vi "Main.vi"() -> ()   [LabVIEW 2019, in "gRPC Scripting Tools.lvlib"]
uses:
  gRPC Scripting Tools.lvlib
  TypeDefs/Project Settings.ctl
panel:
  in  "Generate":enum16{"gRPC Server", "gRPC Client", "Both"}(ring)
  in  "Target Name":string
  in  "Generated Library Name (\"_server\" / \"_client\" will be auto appended)":string
  in  "Target Project":path
  in  "Proto File Path":path
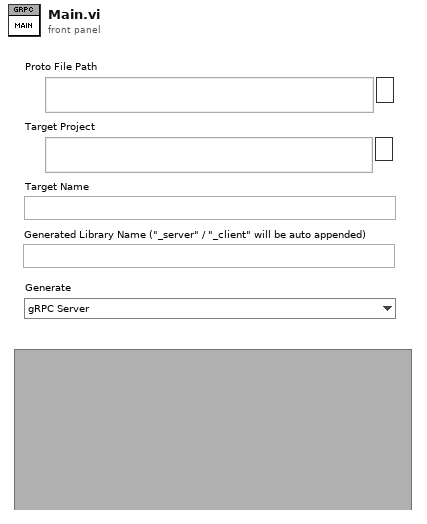
[diagram p1: front panel]
types:
  T1 = typedef "gRPC Scripting Tools.lvlib/RPC Method Parameters.ctl" = cluster{"RPC Method Name":string, "Request Metadata Name":string, "Response Metadata Name":string, "Client Streaming":bool, "Server Streaming":bool}
  T2 = typedef "gRPC Scripting Tools.lvlib/Message Metadata (Scripting).ctl" = cluster{"Version":i32, "Name":string, "Type Url":string, "Elements":T3[]}
  T3 = typedef "gRPC Scripting Tools.lvlib/Message Element Metadata (Scripting).ctl" = cluster{"Field Name":string, "Embedded Message Name":string, "Protobuf Index":i32, "MessageElementType":T4, "Repeated":bool}
  T4 = typedef "gRPC Scripting Tools.lvlib/Message Element Type.ctl" = enum32{"Int32Value", "FloatValue", "DoubleValue", "BoolValue", "StringValue", "MessageValue", "Int64Value", "UInt32Value", "UInt64Value", "EnumValue", "Bytes", "Fixed64", "Fixed32", "SFixed64", "SFixed32", "SInt64", "SInt32"}
  T5 = typedef "gRPC Scripting Tools.lvlib/Project Settings.ctl" = cluster{"Target Project Path":path, "Target Name":string, "Server Name":string, "Library Path":path}
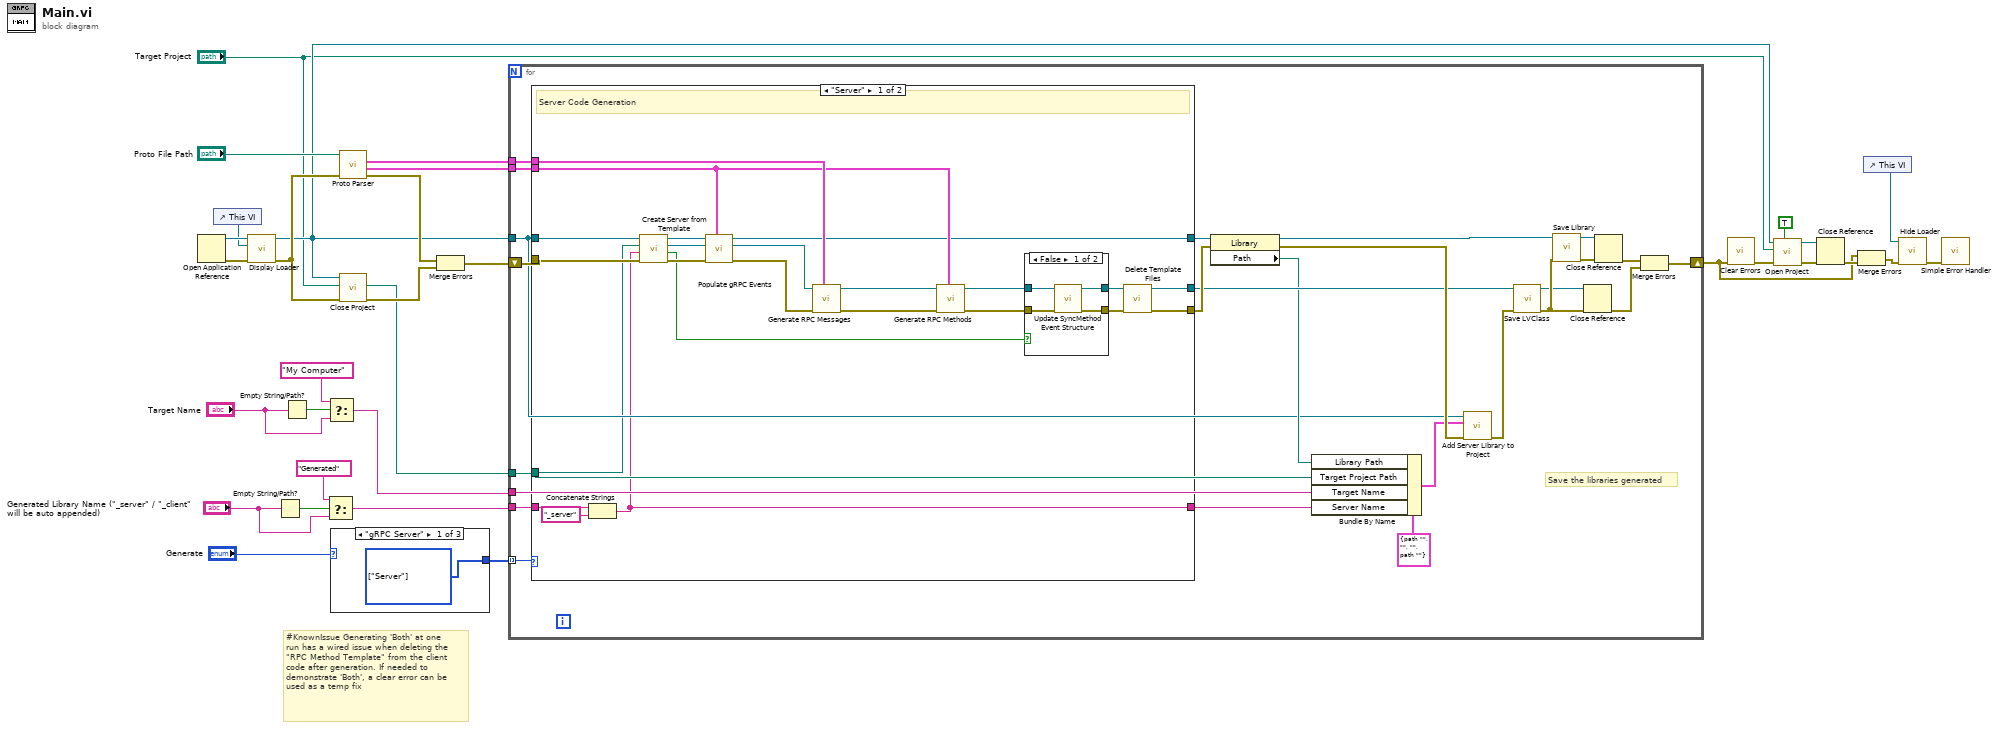
[diagram p0: block diagram]
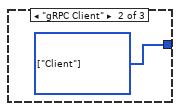
[diagram p2: hidden frame]
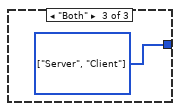
[diagram p3: hidden frame]
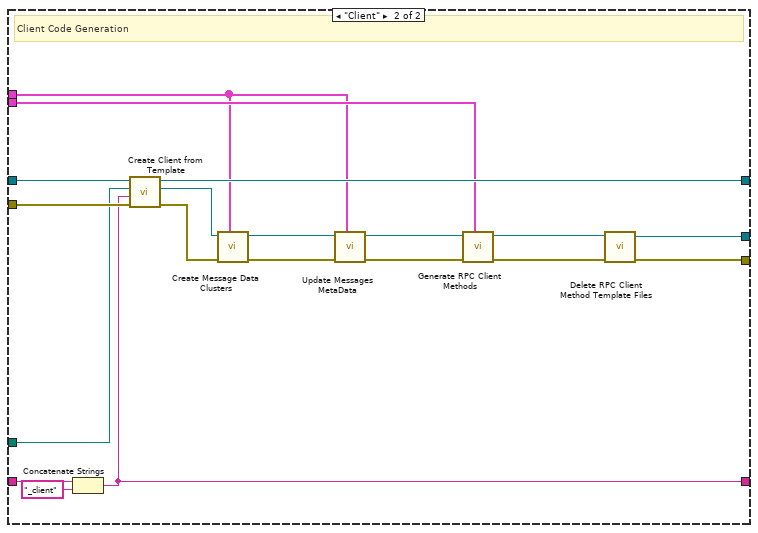
[diagram p5: hidden frame]
diagram:
  # "#KnownIssue Generating 'Both' at one run has a wired issue when deleting the \"RPC Method Template\" from the client code after generation. If needed to demonstrate 'Both', a clear error can be used as a temp fix"
  n1 = Open Application Reference() -> (0:w22:errorcluster, 3:w21:refnum<vi>)  [unwired: 4 in]
  n2 = control-ref of="This VI"() -> (w19:refnum<vi>)
  n3 = call "Display Loader.vi"("error in (no error)"=w22, "VI in"=w19, "application ref in"=w21) -> ("error out"=w20:errorcluster, "application ref out"=w7:refnum<vi>)  [unwired: 7 in]
  n4 = Empty String/Path?(string/path="Generated Library Name (\"_server\" / \"_client\" will be auto appended)") -> (empty?=w32:bool)
  n5 = Empty String/Path?(string/path="Target Name") -> (empty?=w14:bool)
  n6 = Select(t="Generated" ("Path"), s=w32, f="Generated Library Name (\"_server\" / \"_client\" will be auto appended)") -> (s? t:f=w16:string)
  n7 = Select(t="My Computer" ("Path"), s=w14, f="Target Name") -> (s? t:f=w12:string)
  n8 = case shown="\"gRPC Server\"" "Generate" {
    tunnel: [w33 w34 w35] -> w11
    frame "gRPC Server" {
      w33 = enum16{"Server", "Client"}[] [enum."Server"] items=["Server", "Client"]
    }
    frame "gRPC Client" {
      w34 = enum16{"Server", "Client"}[] [enum."Client"] items=["Server", "Client"]
    }
    frame "Both" {
      w35 = enum16{"Server", "Client"}[] [enum."Server", enum."Client"] items=["Server", "Client"]
    }
  }
  n9 = call "Proto Parser.vi"("error in (no error)"=w20, ".proto file path"="Proto File Path") -> ("error out"=w28:errorcluster, "gRPC Method Parameters"=w24:T1[], "gRPC Messages Parameters"=w25:T2[])  [unwired: 7 in]
  n10 = call "Close Project.vi"("error in (no error)"=w20, "Project Path in"="Target Project", "Application reference"=w7) -> ("error out"=w27:errorcluster, "Project Path out"=w17:path)  [unwired: 6 in, 1 out]
  n11 = Merge Errors(w28, w27) -> (w26:errorcluster)
  n12 = for {
    tunnel: w25 -> [w58]
    tunnel: w24 -> [w57]
    tunnel: w17 -> [w37]
    tunnel: w16 -> [w43]
    tunnel: w12 -> [w42]
    tunnel: w7 -> [w39]
    shift-right: [w36] -> w1
    shift-left: w26 -> [w59]
    tunnel: w11 -> [w41] mode=indexing
    # "Save the libraries generated"
    n13 = case shown="\"Server\"" w41 {
      tunnel: w59 -> [w73 w108]
      tunnel: w58 -> [w72 w90]
      tunnel: w57 -> [w71 w99]
      tunnel: w39 -> [w70 w107]
      tunnel: [w69 w102] -> w56
      tunnel: [w66 w96] -> w48
      tunnel: [w65 w95] -> w47
      tunnel: w37 -> [w64 w106]
      tunnel: w43 -> [w63 w105]
      tunnel: [w62 w104] -> w40
      frame "Server" {
        # "Server Code Generation"
        n14 = Concatenate Strings(w63, "_server" ("string")) -> (w62:string)
        n15 = call "Create Server from Template.vi"("error in (no error)"=w73, "Generated Server Name"=w62, "Target Project Path"=w64, "Application ref in"=w70) -> ("error out"=w77:errorcluster, "Already exists ?"=w74:bool, "Server class out"=w80:refnum<vi>, "Server library out"=w81:refnum<vi>)  [unwired: 4 in]
        n16 = call "Populate gRPC Events.vi"("RPC Method Parameters"=w71, "error in (no error)"=w77, "Server class in"=w80, "Server library in"=w81) -> ("error out"=w79:errorcluster, "Server class out"=w78:refnum<vi>, "Server library out"=w69:refnum<vi>)  [unwired: 5 in]
        n17 = call "Generate RPC Messages.vi"("Messages MetaData"=w72, "error in (no error)"=w79, "LVClassLibrary in"=w78) -> ("error out"=w75:errorcluster, "LVClassLibrary out"=w76:refnum<vi>)  [unwired: 7 in]
        n18 = call "Generate RPC Methods.vi"("RPC Method Parameters"=w71, "error in (no error)"=w75, "Server class in"=w76) -> ("error out"=w83:errorcluster, "Server class out"=w82:refnum<vi>)  [unwired: 7 in]
        n19 = case shown="False" w74 {
          tunnel: w83 -> [w87 w88]
          tunnel: w82 -> [w86 w89]
          tunnel: [w85 w88] -> w68
          tunnel: [w84 w89] -> w67
          frame False {
            n20 = call "Update SyncMethod Event Structure.vi"("error in (no error)"=w87, "Server class in"=w86) -> ("error out"=w85:errorcluster, "Server class out"=w84:refnum<vi>)  [unwired: 8 in]
          }
          frame True {
          }
        }
        n21 = call "Delete Template Files.vi"("error in (no error)"=w68, "LVClassLibrary in"=w67) -> ("error out"=w66:errorcluster, "LVClassLibrary out"=w65:refnum<vi>)  [unwired: 8 in]
      }
      frame "Client" {
        # "Client Code Generation"
        n22 = Concatenate Strings(w105, "_client" ("string")) -> (w104:string)
        n23 = call "Create Client from Template.vi"("error in (no error)"=w108, "Generated Server Name"=w104, "Target Project Path"=w106, "Application ref in"=w107) -> ("error out"=w100:errorcluster, "Server class out"=w101:refnum<vi>, "Server library out"=w102:refnum<vi>)  [unwired: 4 in, 1 out]
        n24 = call "Create Message Data Clusters.vi"("Message parameters"=w90, "error in (no error)"=w100, "Server class in"=w101) -> ("error out"=w91:errorcluster, "Server class out"=w94:refnum<vi>)  [unwired: 7 in]
        n25 = call "Update Messages MetaData.vi"("Messages MetaData"=w90, "error in (no error)"=w91, "LVClassLibrary in"=w94) -> ("error out"=w92:errorcluster, "LVClassLibrary out"=w93:refnum<vi>)  [unwired: 7 in]
        n26 = call "Generate RPC Client Methods.vi"("RPC Method Parameters"=w99, "error in (no error)"=w92, "Server class in"=w93) -> ("error out"=w97:errorcluster, "Server class out"=w98:refnum<vi>)  [unwired: 7 in]
        n27 = call "Delete RPC Client Method Template Files.vi"("error in (no error)"=w97, "LVClassLibrary in"=w98) -> ("error out"=w96:errorcluster, "LVClassLibrary out"=w95:refnum<vi>)  [unwired: 8 in]
      }
    }
    n28 = property class="Library"(reference=w56, error in=w48) -> (reference out=w55:refnum<vi>, error out=w52:errorcluster, "Path"=w45:path)
    n29 = Bundle By Name(cluster=T5 {"Target Project Path"=path "", "Target Name"="", "Server Name"="", "Library Path"=path ""} ("Project Settings"), "Library Path"=w45, "Target Project Path"=w37, "Target Name"=w42, "Server Name"=w40) -> (w44:T5)
    n30 = call "Add Server Library to Project.vi"("error in (no error)"=w52, "Project Settings"=w44, "Application in"=w39) -> ("error out"=w38:errorcluster)  [unwired: 8 in]
    n31 = call "Save LVClass.vi"("error in (no error)"=w38, "LVClassLibrary in"=w47) -> ("error out"=w51:errorcluster, "LVClassLibrary out"=w50:refnum<vi>)  [unwired: 8 in]
    n32 = call "Save Library.vi"("error in (no error)"=w51, "Library in"=w55) -> ("error out"=w54:errorcluster, "Library out"=w53:refnum<vi>)  [unwired: 8 in]
    n33 = Close Reference(reference=w50, error in (no error)=w51) -> (error out=w49:errorcluster)
    n34 = Close Reference(reference=w53, error in (no error)=w54) -> (error out=w60:errorcluster)
    n35 = Merge Errors(w60, w49) -> (w36:errorcluster)
  }
  n36 = call <vilib>:"Clear Errors.vi"("error in (no error)"=w1) -> ("error out"=w3:errorcluster)  [unwired: 5 in, 1 out]
  n37 = call "Open Project.vi"("Open Project Window ?"=TRUE, "error in (no error)"=w3, "Project Path in"="Target Project", "Application reference"=w7) -> ("error out"=w5:errorcluster, "Application out"=w6:refnum<vi>)  [unwired: 5 in, 1 out]
  n38 = Close Reference(reference=w6, error in (no error)=w5) -> (error out=w9:errorcluster)
  n39 = Merge Errors(w1, w9) -> (w2:errorcluster)
  n40 = control-ref of="This VI"() -> (w23:refnum<vi>)
  n41 = call "Hide Loader.vi"("error in (no error)"=w2, "VI in"=w23) -> ("error out"=w18:errorcluster)  [unwired: 9 in]
  n42 = call <vilib>:"Simple Error Handler.vi"("error in (no error)"=w18) -> ()  [unwired: 4 in, 5 out]
